vi "GenerateFilter.vi"(8 "error in (no error)":errorcluster, 10 "FFT reference":refnum<vi>, 11 "FFT cluster IN":T1) -> (3 "filter out":dbl[][](array[numeric]))   [LabVIEW 2018, in "Photon Filtering.lvlib"]
uses:
  Photon Filtering.lvlib
  <vilib>/Analysis/baseanly.llb/Real Outer Product.vi
  <vilib>/Analysis/Matrix/Numeric/Conversions/Matrix To Array - RM.vi
  <vilib>/Analysis/NI_AALBase.lvlib
  <vilib>/Analysis/Matrix/NI_Matrix.lvlib
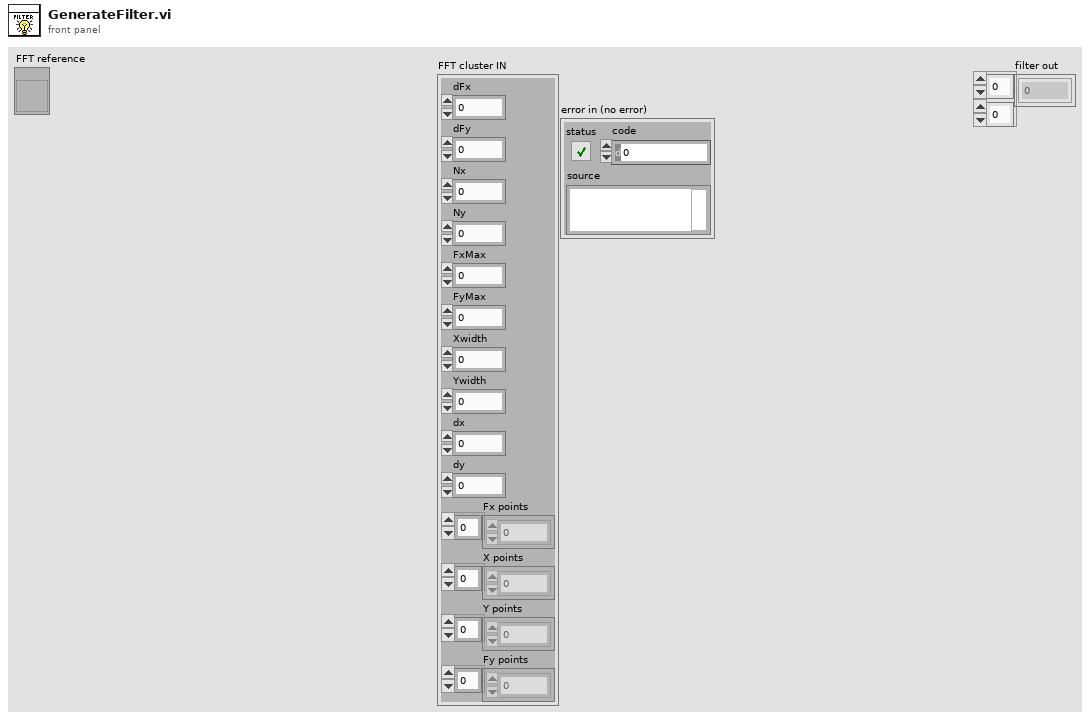
[diagram p1: front panel]
types:
  T1 = cluster{"dFx":dbl, "dFy":dbl, "Nx":i32, "Ny":i32, "FxMax":dbl, "FyMax":dbl, "Xwidth":dbl, "Ywidth":dbl, "dx":dbl, "dy":dbl, "Fx points":dbl[], "X points":dbl[], "Y points":dbl[], "Fy points":dbl[]}
  T2 = typedef "NI_Matrix.lvlib/RealMatrix.ctl" = dbl[][]
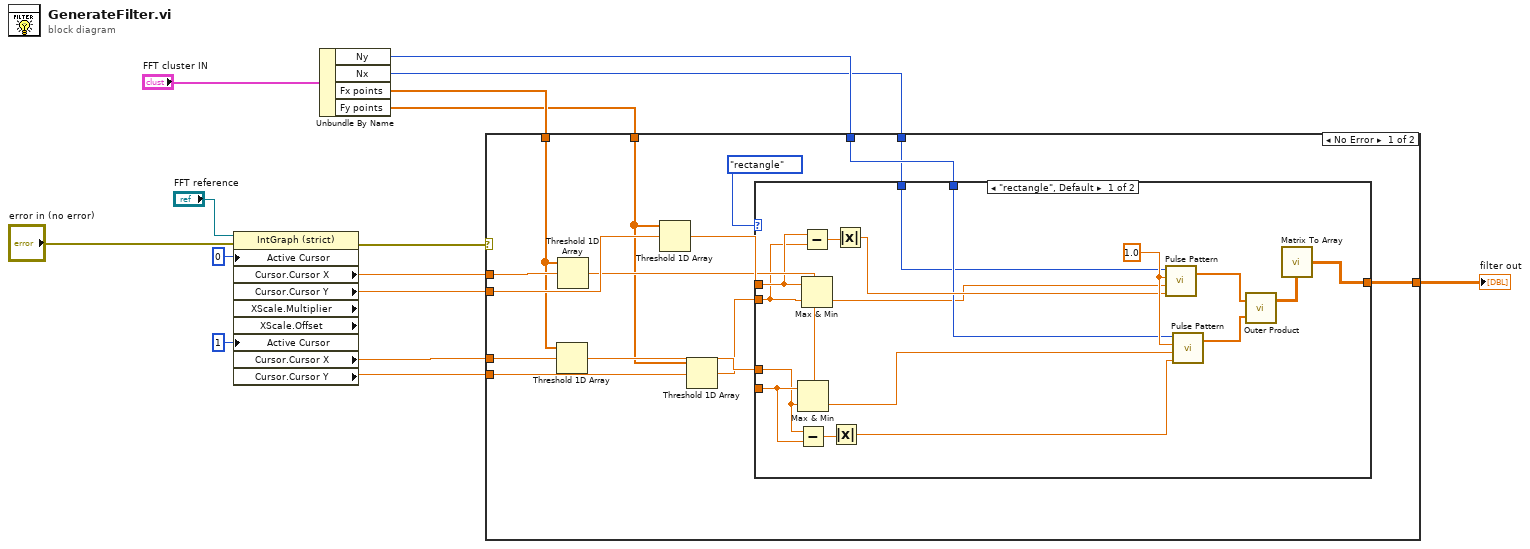
[diagram p0: block diagram]
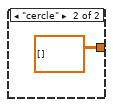
[diagram p2: hidden frame]
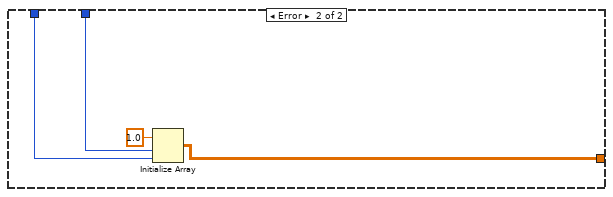
[diagram p3: hidden frame]
diagram:
  n1 = property class="IntGraph (strict)" props=["Active Cursor", "Cursor", "Cursor X", "Cursor", "Cursor Y", "XScale", "Multiplier", "XScale", "Offset", "Active Cursor", "Cursor", "Cursor X", "Cursor", "Cursor Y"](reference="FFT reference", error in="error in (no error)", "Active Cursor"=u32 0, "Active Cursor"=u32 1) -> (error out=w1:errorcluster, "Cursor.Cursor X"=w12:dbl, "Cursor.Cursor Y"=w10:dbl, "Cursor.Cursor X"=w11:dbl, "Cursor.Cursor Y"=w9:dbl)  [unwired: 3 out]
  n2 = Unbundle By Name("FFT cluster IN") -> ("Ny"=w5:i32, "Nx"=w4:i32, "Fx points"=w8:dbl[], "Fy points"=w7:dbl[])
  n3 = case shown="No Error" w1 {
    tunnel: w12 -> [w28 _]
    tunnel: w11 -> [w27 _]
    tunnel: w10 -> [w25 _]
    tunnel: w9 -> [w23 _]
    tunnel: w8 -> [w20 _]
    tunnel: w7 -> [w19 _]
    tunnel: w5 -> [w18 w50]
    tunnel: w4 -> [w17 w51]
    tunnel: [w16 w48] -> w3
    frame No Error {
      n4 = Threshold 1D Array(2:w27, 3:w20) -> (0:w26:dbl)  [unwired: 1 in]
      n5 = Threshold 1D Array(2:w28, 3:w20) -> (0:w21:dbl)  [unwired: 1 in]
      n6 = Threshold 1D Array(2:w25, 3:w19) -> (0:w24:dbl)  [unwired: 1 in]
      n7 = Threshold 1D Array(2:w23, 3:w19) -> (0:w22:dbl)  [unwired: 1 in]
      n8 = case shown="\"rectangle\", Default" enum16{"rectangle", "cercle"}."rectangle" {
        tunnel: [w44 dbl[][] [] ("Real 2D Array")] -> w16
        tunnel: w18 -> [w38 _]
        tunnel: w17 -> [w37 _]
        tunnel: w24 -> [w35 _]
        tunnel: w22 -> [w34 _]
        tunnel: w21 -> [w33 _]
        tunnel: w26 -> [w30 _]
        frame "rectangle", Default {
          w46 = 1.0 ("amplitude")
          n9 = Max & Min(x=w33, y=w30) -> (min(x,y)=w40:dbl)  [unwired: 1 out]
          n10 = Subtract(x=w30, y=w33) -> (x-y=w41:dbl)
          n11 = Subtract(x=w35, y=w34) -> (x-y=w43:dbl)
          n12 = Max & Min(x=w35, y=w34) -> (min(x,y)=w36:dbl)  [unwired: 1 out]
          n13 = Absolute Value(x=w41) -> (abs(x)=w32:dbl)
          n14 = Absolute Value(x=w43) -> (abs(x)=w42:dbl)
          n15 = call <vilib>:"Pulse Pattern.vi"("width"=w42, "delay"=w36, "amplitude"=w46, "samples"=w37) -> ("Pulse Pattern"=w31:dbl[])  [unwired: 1 out]
          n16 = call <vilib>:"Pulse Pattern.vi"("width"=w32, "delay"=w40, "amplitude"=w46, "samples"=w38) -> ("Pulse Pattern"=w39:dbl[])  [unwired: 1 out]
          n17 = call-poly <vilib>:"Outer Product.vi"("Y Vector"=w39, "X Vector"=w31) -> ("Outer Product"=w45:T2)  [unwired: 1 out]
          n18 = call-poly <vilib>:"Matrix To Array.vi"("Real Matrix"=w45) -> ("Real 2D Array"=w44:dbl[][])
        }
        frame "cercle" {
        }
      }
    }
    frame Error {
      n19 = Initialize Array(1.0 ("element"), w51, w50) -> (w48:dbl[][])
    }
  }
  "filter out" <- w3
